vi "Create Antinodesvi.vi"(10 "Antena 2":T1, 11 "Antena 1":T1) -> (2 "AntiNode 2 Out":T1, 3 "AntiNoed 1 Out":T1)   [LabVIEW 2024]
uses:
  Cluster_Position.ctl
panel:
  in  "Max Grid Index":T1
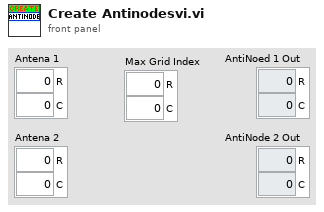
[diagram p1: front panel]
types:
  T1 = typedef "Cluster_Position.ctl" = cluster{"R":i32, "C":i32}
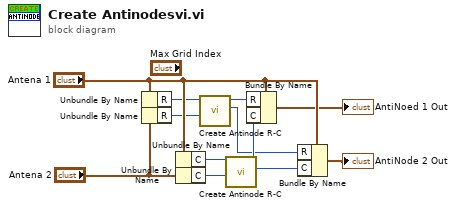
[diagram p0: block diagram]
diagram:
  n1 = Unbundle By Name("Antena 1") -> ("R"=w8:i32)
  n2 = Unbundle By Name("Antena 2") -> ("R"=w9:i32)
  n3 = Unbundle By Name("Antena 1") -> ("C"=w10:i32)
  n4 = Unbundle By Name("Antena 2") -> ("C"=w11:i32)
  n5 = call "Create Antinode R-C.vi"("2"=w9, "1"=w8) -> ("Antinode 2"=w1:i32, "Antinode 1"=w4:i32)  [unwired: 8 in]
  n6 = call "Create Antinode R-C.vi"("2"=w11, "1"=w10) -> ("Antinode 2"=w2:i32, "Antinode 1"=w3:i32)  [unwired: 8 in]
  n7 = Bundle By Name(cluster="Antena 1", "R"=w4, "C"=w3) -> (→"AntiNoed 1 Out":T1)
  n8 = Bundle By Name(cluster="Antena 1", "R"=w1, "C"=w2) -> (→"AntiNode 2 Out":T1)
